vi "Read Attributes.vi"(11 "Launch Guest Manager Msg":refnum<class "Launch Guest Manager Msg.lvclass">) -> (2 "Payload":cluster{"Check-in":bool})   [LabVIEW 2023, in "Rooms Manager UI.lvlib" / "Launch Guest Manager Msg.lvclass"]
uses:
  Launch Guest Manager Msg.lvclass
  Launch Guest Manager Msg.lvclass/Launch Guest Manager Msg.ctl
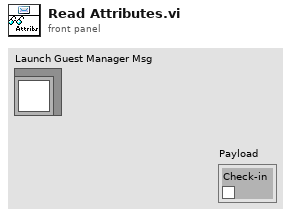
[diagram p1: front panel]
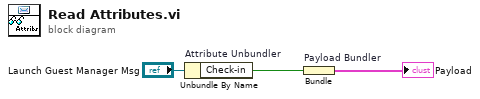
[diagram p0: block diagram]
diagram:
  n1 = Unbundle By Name "Attribute Unbundler"("Launch Guest Manager Msg") -> ("Check-in"=w1:bool)
  n2 = Bundle "Payload Bundler"("Check-in"=w1) -> (→"Payload":cluster{"Check-in":bool})  [unwired: 1 in]
